vi "Rover_main.vi"() -> ()   [LabVIEW 2018]
uses:
  <vilib>/sound2/lvsound2.llb/Sound File Read Open.vi
  <vilib>/Instr/_visa.llb/VISA Configure Serial Port (Instr).vi
  <vilib>/Utility/file.llb/Write Delimited Spreadsheet (string).vi
  <vilib>/Utility/inputDevices.llb/keyboardAcquire.vi
  <vilib>/Utility/inputDevices.llb/closeKeyboard.vi
  <resource>/objmgr/imaqdx.rc
  <vilib>/vision/driver/NI_Vision_Acquisition_Software.lvlib
panel:
  out "DIS":dbl(knob) scale=0.0..500.0
  in  "Frames Per Second":u32=9
  out "Right view":bool
  out "Left view":bool
  out "Front view":bool
  in  "Camera port":refnum<k21>="cam5" caption="IMAQdx Session"
  in  "Video Modes":i32(listbox)
  out "Image":T1(plugin-control)
  out "AIR":dbl(knob) scale=500.0..1300.0
  out "Air Pressure Monitoring":string
  in  "path 3":path=path "C:/Users/向成/Desktop/ROVER PROJECT/LABVIEW codes/voice recognition/danger.wav" caption="路径"
  out "Voice recognition":bool
  in  "path":path=path "C:/Users/向成/Desktop/ROVER PROJECT/LABVIEW codes/voice recognition/activated.wav" caption="路径"
  in  "path 2":path=path "C:/Users/向成/Desktop/ROVER PROJECT/LABVIEW codes/voice recognition/failed.wav" caption="路径"
  out "Distance Monitoring":string
  in  "Sensors activation":bool
  out "TEM":dbl(slide) caption="量表" scale=0.0..50.0
  out "Temperature Monitoring":string
  out "gear":dbl(slide) scale=0.0..3.0
  out "LEFT":bool
  out "RIGHT":bool
  out "UP":bool
  out "DOWN":bool
  out "字符串监控":string
  in  "?":bool
  in  "Serial port":refnum<visa-resource-name>="COM4"
  # "Gear Stick Control"
  # "Motors Control"
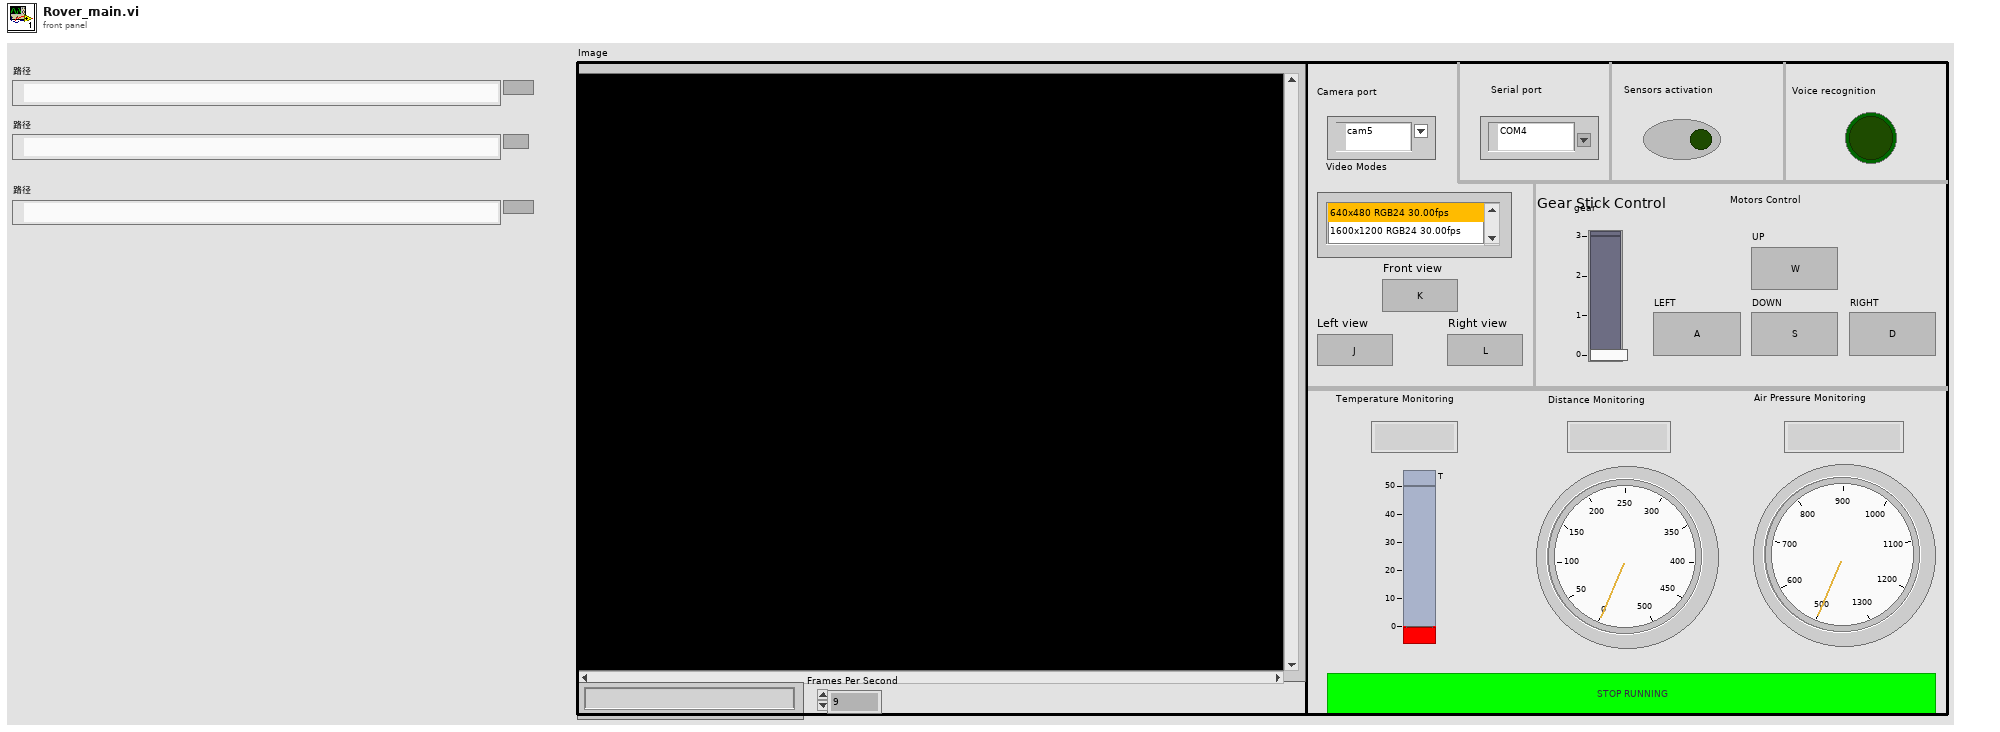
[diagram p1: front panel]
types:
  T1 = typedef "IMAQ Image.ctl" = refnum<image>
  T2 = enum16{"0", "1", "2", "3", "4", "5", "6", "7", "8", "9", "A", "B", "C", "D", "E", "F", "G", "H", "I", "J", "K", "L", "M", "N", "O", "P", "Q", "R", "S", "T", "U", "V", "W", "X", "Y", "Z", "F1", "F2", "F3", "F4", "F5", "F6", "F7", "F8", "F9", "F10", "F11", "F12", "F13", "F14", "F15", "ADD", "BACK", "BACKSLASH", "CAPITAL", "COMMA", "DECIMAL", "DELETE", "DIVIDE", "DOWN", "END", "EQUALS", "ESCAPE", "GRAVE (`)", "HOME", "INSERT", "LBRACKET", "LCONTROL", "LEFT", "L ALT", "LSHIFT", "LWIN", "MINUS", "MULTIPLY", "NEXT", "NUMLOCK", "NUMPAD_0", "NUMPAD_1", "NUMPAD_2", "NUMPAD_3", "NUMPAD_4", "NUMPAD_5", "NUMPAD_6", "NUMPAD_7", "NUMPAD_8", "NUMPAD_9", "PAUSE", "PERIOD", "PRIOR (PG UP)", "RBRACKET", "RCONTROL", "RETURN", "RIGHT", "R ALT", "RSHIFT", "RWIN", "SCROLL", "SEMICOLON", "SLASH", "SPACE", "SUBTRACT", "TAB", "UP", "ENTER (num pad)", "' (quote)"}
  T3 = typedef "Sound File Refnum.ctl" = refnum<file>
  T4 = enum32{"existing file", "new file", "new or existing file", "existing dir", "new dir", "new or existing dir", "existing file (use LLBs)", "new file (use LLBs)", "new or existing file (use LLBs)", "new or existing file or directory (use LLBs)"}
  T5 = typedef "IMAQdx.ctl" = refnum<k21>
  T6 = typedef "AviRefnum.ctl" = refnum<k1>
  T7 = enum16{"0", "1", "2", "3", "4", "5", "6", "7", "8", "9", "A", "B", "C", "D", "E", "F", "G", "H", "I", "J", "K", "L", "M", "N", "O", "P", "Q", "R", "S", "T", "U", "V", "W", "X", "Y", "Z", "F1", "F2", "F3", "F4", "F5", "F6", "F7", "F8", "F9", "F10", "F11", "F12", "F13", "F14", "F15", "ADD", "BACK", "BACKSLASH", "CAPITAL", "COMMA", "DECIMAL", "DELETE", "DIVIDE", "DOWN", "END", "EQUALS", "ESCAPE", "GRAVE (`)", "HOME", "INSERT", "LBRACKET", "LCONTROL", "LEFT", "L ALT", "LSHIFT", "LWIN", "MINUS", "MULTIPLY", "NEXT", "NUMLOCK", "NUMPAD_0", "NUMPAD_1", "NUMPAD_2", "NUMPAD_3", "NUMPAD_4", "NUMPAD_5", "NUMPAD_6", "NUMPAD_7", "NUMPAD_8", "NUMPAD_9", "PAUSE", "PERIOD", "PRIOR (PG UP)", "RBRACKET", "RCONTROL", "RETURN", "RIGHT", "R ALT", "RSHIFT", "RWIN", "SCROLL", "SEMICOLON", "SLASH", "SPACE", "SUBTRACT", "TAB", "UP", "ENTER (num pad)", "' (quote)"}[]
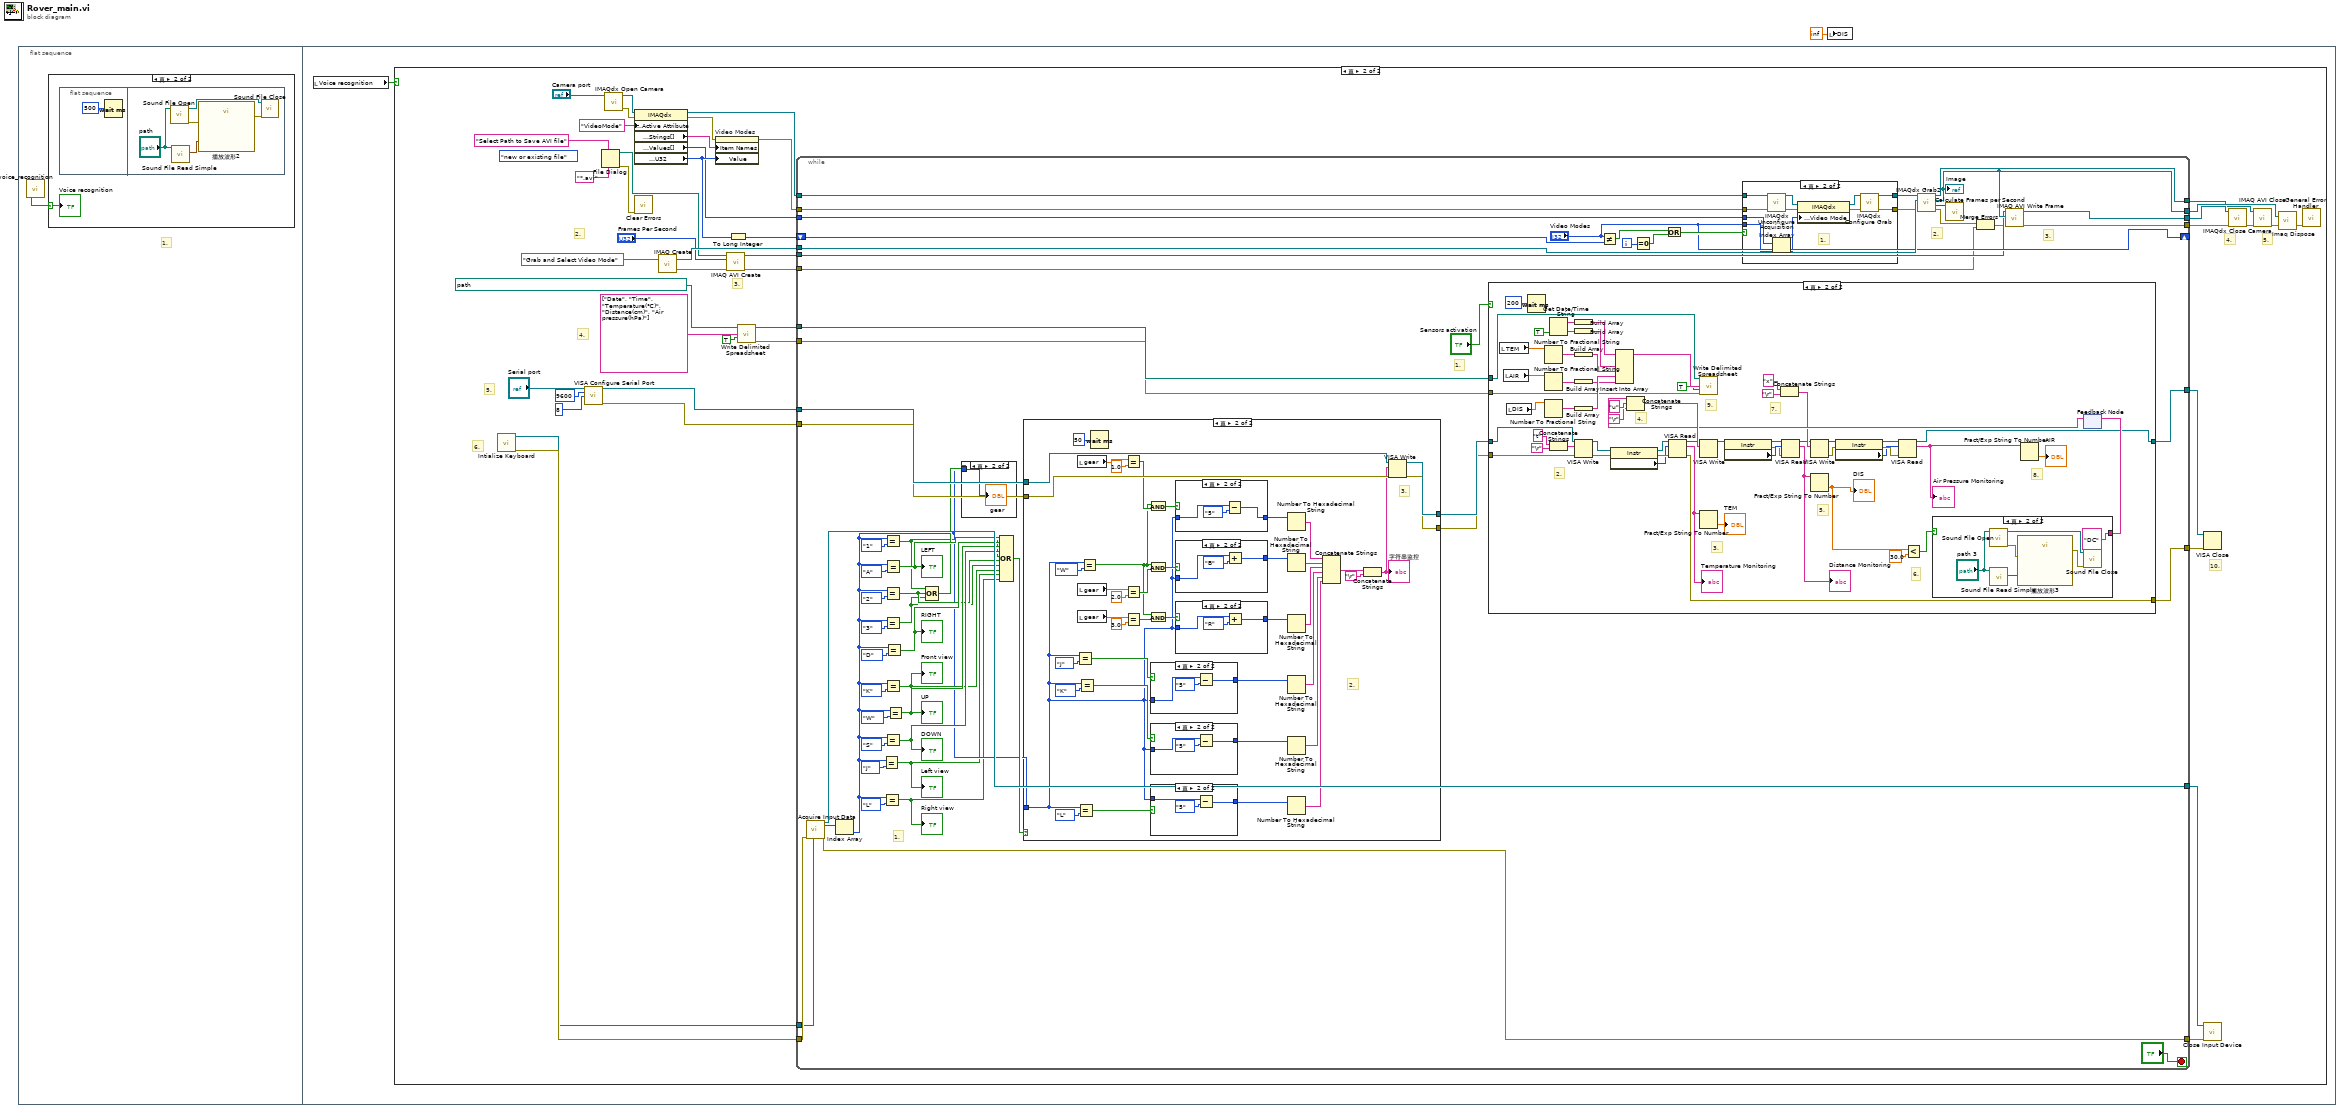
[diagram p0: block diagram]
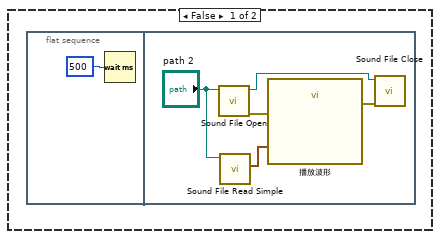
[diagram p2: hidden frame]
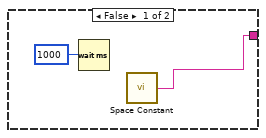
[diagram p6: hidden frame]
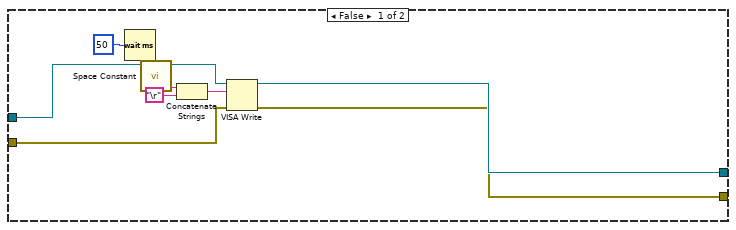
[diagram p8: hidden frame]
diagram:
  n1 = flat-sequence {
    frame #0 {
      # "1."
      n2 = call "voice_recognition.vi"() -> ("x < y?"=w2:bool)  [unwired: 5 in, 10 out]
      n3 = case shown="真" w2 {
        selector: w2 -> [_ w9]
        frame False {
          n4 = flat-sequence {
            frame #0 {
              n5 = Wait (ms)(milliseconds to wait=u32 500 ("等待时间（毫秒）")) -> ()  [unwired: 1 out]
            }
            frame #1 {
              n6 = call-poly <vilib>:"Sound File Open.vi"("path"="path 2") -> ("error out"=w5:errorcluster, "sound file refnum"=w7:T3)  [unwired: 9 in]
              n7 = call <vilib>:"Sound File Read Simple.vi"("path"="path 2") -> ("data"=w6:waveform(dbl)[])  [unwired: 7 in, 3 out]
              n8 = call "播放波形"("Data"=w6, "error in"=w5) -> ("error out"=w4:errorcluster)  [unwired: 17 in]
              n9 = call <vilib>:"Sound File Close.vi"("error in (no error)"=w4, "sound file refnum"=w7) -> ()  [unwired: 9 in, 1 out]
            }
          }
        }
        frame True {
          n10 = flat-sequence {
            frame #0 {
              n11 = Wait (ms)(milliseconds to wait=u32 500 ("等待时间（毫秒）")) -> ()  [unwired: 1 out]
            }
            frame #1 {
              n12 = call-poly <vilib>:"Sound File Open.vi"("path"="path") -> ("error out"=w13:errorcluster, "sound file refnum"=w11:T3)  [unwired: 9 in]
              n13 = call <vilib>:"Sound File Read Simple.vi"("path"="path") -> ("data"=w12:waveform(dbl)[])  [unwired: 7 in, 3 out]
              n14 = call "播放波形2"("Data"=w12, "error in"=w13) -> ("error out"=w14:errorcluster)  [unwired: 17 in]
              n15 = call <vilib>:"Sound File Close.vi"("error in (no error)"=w14, "sound file refnum"=w11) -> ()  [unwired: 9 in, 1 out]
            }
          }
          "Voice recognition" <- w9
        }
      }
    }
    frame #1 {
      n16 = local read "Voice recognition"() -> (w16:bool)
      n17 = case shown="真" w16 {
        frame False {
        }
        frame True {
          (unwired) T4."new or existing file" ("select mode (2)")
          # "10."
          # "5."
          # "4."
          # "6."
          # "3."
          # "5."
          # "4."
          # "2."
          n18 = call <vilib>:"Intialize Keyboard.vi"() -> ("error out"=w54:errorcluster, "device ID"=w53:refnum<k1>)  [unwired: 10 in]
          n19 = call-poly "VISA Configure Serial Port"("VISA resource name"="Serial port", "baud rate (9600)"=u32 9600, "data bits (8)"=u16 8) -> ("VISA resource name out"=w58:refnum<visa-resource-name>, "error out"=w59:errorcluster)  [unwired: 3 in, 8 out]
          n20 = File Dialog(6:"*.avi" ("pattern"), 7:"Select Path to Save AVI file" ("prompt")) -> (0:w18:errorcluster, 3:w19:path)  [unwired: 1 in, 6 out]
          n21 = call <vilib>:"IMAQdx Open Camera.vi"("Session In"="Camera port") -> ("error out"=w47:errorcluster, "Session Out"=w46:T5)  [unwired: 2 in, 7 out]
          n22 = property class="IMAQdx"(reference=w46, error in=w47, "Camera Attributes:Active Attribute"="VideoMode" ("ActiveAttribute")) -> (reference out=w40:T5, error out=w48:errorcluster, "Camera Attributes:Enum:Strings[]"=w49:string[], "Camera Attributes:Enum:Values[]"=w42:u32[], "Camera Attributes:Value:U32"=w50:u32)
          n23 = call <vilib>:"Clear Errors.vi"("error in (no error)"=w18) -> ()  [unwired: 5 in, 2 out]
          n24 = call "IMAQ Create"("Image Name"="Grab and Select Video Mode") -> ("New Image"=w41:T1, "error out"=w24:errorcluster)  [unwired: 3 in, 1 out]
          n25 = property on="Video Modes" class="LstBox (严格)"(error in=w48, "Item Names"=w49, "Value"=w50) -> (error out=w25:errorcluster)  [unwired: 1 in, 1 out]
          n26 = call "IMAQ AVI Create"("error in (no error)"=w24, "Frames Per Second"="Frames Per Second", "AVI Path"=w19) -> ("error out"=w17:errorcluster, "Avi Refnum"=w23:T6)  [unwired: 4 in, 3 out]
          n27 = To Long Integer(number=w50) -> (32bit integer=w39:i32)
          n28 = call-poly <vilib>:"Write Delimited Spreadsheet.vi"("file path (dialog if empty)"=path "C:/Users/向成/Desktop/rover_project/Data_Storage/data_acquired", "1D data"=string[] ["Date", "Time", "Temperature(℃)", "Distance(cm)", "Air pressure(hPa)"], "append to file? (new file:F)"=TRUE) -> ("new file path (Not A Path if cancelled)"=w31:path, "error out"=w30:errorcluster)  [unwired: 11 in]
          n29 = while {
            tunnel: w53 -> [w118]
            tunnel: w54 -> [w119]
            tunnel: w58 -> [w116]
            tunnel: w59 -> [w115]
            tunnel: [w117] -> w56
            tunnel: [w114] -> w57
            tunnel: [w96] -> w60
            tunnel: w42 -> [w93]
            tunnel: w41 -> [w92]
            tunnel: w40 -> [w91]
            shift-right: ["Video Modes"] -> _
            shift-left: w39 -> [w83]
            tunnel: [w67] -> w37
            tunnel: [w64] -> w36
            tunnel: [w82] -> w35
            tunnel: w31 -> [w71]
            tunnel: w30 -> [w70]
            tunnel: [w69] -> w29
            tunnel: w25 -> [w68]
            tunnel: [w66] -> w28
            tunnel: w23 -> [w65]
            tunnel: w17 -> [w62]
            i -> [w81]
            stop <- "?" stop-if-true
            # "1."
            # "3."
            # "2."
            # "1."
            n30 = call-poly <vilib>:"Acquire Input Data.vi"("device ID"=w118, "error in (no error)"=w119) -> ("device ID"=w117:refnum<k1>, "keys pressed"=w111:T7, "error out"=w114:errorcluster)  [unwired: 15 in]
            n31 = Index Array(array=w111) -> (element=w75:T2)  [unwired: 1 in]
            n32 = Equal?(x=w75, y=T2."J") -> (x = y?=w74:bool)
            "Left view" <- w74
            n33 = Equal?(x=w75, y=T2."L") -> (x = y?=w73:bool)
            "Right view" <- w73
            n34 = Equal?(x=w75, y=T2."1") -> (x = y?=w99:bool)
            n35 = Equal?(x=w75, y=T2."2") -> (x = y?=w98:bool)
            n36 = Equal?(x=w75, y=T2."3") -> (x = y?=w97:bool)
            n37 = Equal?(x=w75, y=T2."S") -> (x = y?=w101:bool)
            "DOWN" <- w101
            n38 = Equal?(x=w75, y=T2."A") -> (x = y?=w104:bool)
            "LEFT" <- w104
            n39 = Equal?(x=w75, y=T2."K") -> (x = y?=w78:bool)
            "Front view" <- w78
            n40 = Equal?(x=w75, y=T2."D") -> (x = y?=w103:bool)
            "RIGHT" <- w103
            n41 = Equal?(x=w75, y=T2."W") -> (x = y?=w102:bool)
            "UP" <- w102
            n42 = Compound Arithmetic op=OR ("复合运算")(w99, w98, w97) -> (w100:bool)
            n43 = case shown="真" w100 {
              tunnel: w75 -> [_ w201]
              frame False {
              }
              frame True {
                "gear" <- w201
              }
            }
            n44 = Compound Arithmetic op=OR ("复合运算")(w104, w103, w102, w101, w99, w98, w97, w78, w74, w73) -> (w110:bool)
            n45 = case shown="真" w110 {
              tunnel: [w204 w249] -> w95
              tunnel: [w203 w248] -> w94
              tunnel: w75 -> [_ w213]
              tunnel: w116 -> [w205 w247]
              tunnel: w115 -> [w206 w246]
              frame False {
                n46 = Wait (ms)(milliseconds to wait=u32 50 ("等待时间（毫秒）")) -> ()  [unwired: 1 out]
                n47 = call <vilib>:"Space Constant.vi"() -> ("String"=w207:string)
                n48 = Concatenate Strings(w207, "\r") -> (w209:string)
                n49 = VISA Write(VISA resource name=w205, write buffer=w209, error in (no error)=w206) -> (VISA resource name out=w204:refnum<visa-resource-name>, error out=w203:errorcluster)  [unwired: 1 out]
              }
              frame True {
                # "3."
                # "2."
                n50 = Equal?(x=w213, y=T2."J") -> (x = y?=w219:bool)
                n51 = Equal?(x=w213, y=T2."L") -> (x = y?=w217:bool)
                n52 = local read "gear"() -> (w244:dbl)
                n53 = local read "gear"() -> (w238:dbl)
                n54 = local read "gear"() -> (w233:dbl)
                n55 = Equal?(x=w213, y=T2."K") -> (x = y?=w218:bool)
                n56 = Equal?(x=w213, y=T2."W") -> (x = y?=w225:bool)
                n57 = Wait (ms)(milliseconds to wait=u32 50 ("等待时间（毫秒）")) -> ()  [unwired: 1 out]
                n58 = Equal?(x=w244, y=1.0) -> (x = y?=w242:bool)
                n59 = Equal?(x=w238, y=2.0) -> (x = y?=w236:bool)
                n60 = Equal?(x=w233, y=3.0) -> (x = y?=w234:bool)
                n61 = And(x=w225, y=w242) -> (x .and. y?=w241:bool)
                n62 = And(x=w225, y=w236) -> (x .and. y?=w240:bool)
                n63 = And(x=w225, y=w234) -> (x .and. y?=w226:bool)
                n64 = case shown="真" w219 {
                  tunnel: [_ w258] -> w216
                  tunnel: w213 -> [_ w257]
                  frame False {
                  }
                  frame True {
                    n65 = Subtract(x=w257, y=T2."5") -> (x-y=w258:u16)
                  }
                }
                n66 = case shown="真" w218 {
                  tunnel: [_ w255] -> w215
                  tunnel: w213 -> [_ w254]
                  frame False {
                  }
                  frame True {
                    n67 = Subtract(x=w254, y=T2."5") -> (x-y=w255:u16)
                  }
                }
                n68 = case shown="真" w217 {
                  tunnel: [_ w252] -> w214
                  tunnel: w213 -> [_ w251]
                  frame False {
                  }
                  frame True {
                    n69 = Subtract(x=w251, y=T2."5") -> (x-y=w252:u16)
                  }
                }
                n70 = case shown="真" w241 {
                  tunnel: w213 -> [w266 w269]
                  tunnel: [w266 w267] -> w239
                  frame False {
                  }
                  frame True {
                    n71 = Subtract(x=w269, y=T2."5") -> (x-y=w267:u16)
                  }
                }
                n72 = case shown="真" w240 {
                  tunnel: [_ w264] -> w232
                  tunnel: w213 -> [_ w263]
                  frame False {
                  }
                  frame True {
                    n73 = Add(x=w263, y=T2."B") -> (x+y=w264:u16)
                  }
                }
                n74 = case shown="真" w226 {
                  tunnel: [_ w261] -> w229
                  tunnel: w213 -> [_ w260]
                  frame False {
                  }
                  frame True {
                    n75 = Add(x=w260, y=T2."R") -> (x+y=w261:u16)
                  }
                }
                n76 = Number To Hexadecimal String(2:w239) -> (0:w230:string)  [unwired: 1 in]
                n77 = Number To Hexadecimal String(2:w232) -> (0:w231:string)  [unwired: 1 in]
                n78 = Number To Hexadecimal String(2:w229) -> (0:w228:string)  [unwired: 1 in]
                n79 = Number To Hexadecimal String(2:w216) -> (0:w212:string)  [unwired: 1 in]
                n80 = Number To Hexadecimal String(2:w215) -> (0:w210:string)  [unwired: 1 in]
                n81 = Number To Hexadecimal String(2:w214) -> (0:w211:string)  [unwired: 1 in]
                n82 = Concatenate Strings(w230, w231, w228, w212, w210, w211) -> (w227:string)
                n83 = Concatenate Strings(w227, "\r") -> (w224:string)
                "字符串监控" <- w224
                n84 = VISA Write(VISA resource name=w247, write buffer=w224, error in (no error)=w246) -> (VISA resource name out=w249:refnum<visa-resource-name>, error out=w248:errorcluster)  [unwired: 1 out]
              }
            }
            n85 = case shown="真" "Sensors activation" {
              tunnel: [w134 w192] -> w96
              tunnel: w95 -> [w133 w191]
              tunnel: w94 -> [w134 w190]
              tunnel: w71 -> [_ w175]
              tunnel: w70 -> [_ w173]
              tunnel: [w133 w137] -> w69
              frame False {
              }
              frame True {
                # "8."
                # "7."
                # "4."
                # "6."
                # "5."
                # "3."
                # "2."
                # "9."
                n86 = local read "TEM"() -> (w189:dbl)
                n87 = local read "AIR"() -> (w187:dbl)
                n88 = local read "DIS"() -> (w135:dbl)
                n89 = Wait (ms)(milliseconds to wait=u32 200 ("等待时间（毫秒）")) -> ()  [unwired: 1 out]
                n90 = Number To Fractional String(number=w189) -> (F-format string=w188:string)  [unwired: 3 in]
                n91 = Number To Fractional String(number=w187) -> (F-format string=w186:string)  [unwired: 3 in]
                n92 = Number To Fractional String(number=w135) -> (F-format string=w185:string)  [unwired: 3 in]
                n93 = Get Date/Time String(want seconds? (F)=TRUE ("需要秒？(F)")) -> (date string=w179:string, time string=w180:string)  [unwired: 2 in]
                n94 = Concatenate Strings("t" ("字符串"), "\r") -> (w167:string)
                n95 = Build Array(w179) -> (w181:string[])
                n96 = Build Array(w180) -> (w182:string[])
                n97 = Build Array(w188) -> (w184:string[])
                n98 = Build Array(w186) -> (w177:string[])
                n99 = Build Array(w185) -> (w178:string[])
                n100 = VISA Write(VISA resource name=w191, write buffer=w167, error in (no error)=w190) -> (VISA resource name out=w169:refnum<visa-resource-name>, error out=w168:errorcluster)  [unwired: 1 out]
                n101 = property class="Instr"(reference=w169, error in=w168) -> (reference out=w172:refnum<visa-resource-name>, error out=w171:errorcluster, "Serial Settings:Number of Bytes at Serial Port"=w170:u32)
                n102 = Insert Into Array(array=w181, new element #1=w182, new element #2=w184, new element #3=w178, new element #4=w177) -> (w183:string[])  [unwired: 1 in]
                n103 = VISA Read(VISA resource name=w172, byte count=w170, error in (no error)=w171) -> (VISA resource name out=w154:refnum<visa-resource-name>, read buffer=w162:string, error out=w192:errorcluster)  [unwired: 1 out]
                "Temperature Monitoring" <- w162
                n104 = call-poly <vilib>:"Write Delimited Spreadsheet.vi"("file path (dialog if empty)"=w175, "1D data"=w183, "append to file? (new file:F)"=TRUE, "error in (no error)"=w173) -> ()  [unwired: 10 in, 2 out]
                n105 = Fract/Exp String To Number(string=w162) -> (number=→"TEM":dbl)  [unwired: 3 in, 1 out]
                n106 = Concatenate Strings("x" ("字符串"), "\r") -> (w143:string)
                n107 = feedback #1() -> (w149:string)  [unwired: 1 in]
                n108 = Concatenate Strings(w149, "u" ("字符串"), "\r") -> (w159:string)
                n109 = VISA Write(VISA resource name=w154, write buffer=w159) -> (VISA resource name out=w155:refnum<visa-resource-name>)  [unwired: 1 in, 2 out]
                n110 = property class="Instr"(reference=w155) -> (reference out=w156:refnum<visa-resource-name>, error out=w157:errorcluster, "Serial Settings:Number of Bytes at Serial Port"=w158:u32)  [unwired: 1 in]
                n111 = VISA Read(VISA resource name=w156, byte count=w158, error in (no error)=w157) -> (VISA resource name out=w139:refnum<visa-resource-name>, read buffer=w150:string)  [unwired: 2 out]
                "Distance Monitoring" <- w150
                n112 = VISA Write(VISA resource name=w139, write buffer=w143) -> (VISA resource name out=w145:refnum<visa-resource-name>, error out=w144:errorcluster)  [unwired: 1 in, 1 out]
                n113 = Fract/Exp String To Number(string=w150) -> (number=w136:dbl)  [unwired: 3 in, 1 out]
                "DIS" <- w136
                n114 = property class="Instr"(reference=w145, error in=w144) -> (reference out=w148:refnum<visa-resource-name>, error out=w147:errorcluster, "Serial Settings:Number of Bytes at Serial Port"=w146:u32)
                n115 = VISA Read(VISA resource name=w148, byte count=w146, error in (no error)=w147) -> (VISA resource name out=w137:refnum<visa-resource-name>, read buffer=w138:string)  [unwired: 2 out]
                "Air Pressure Monitoring" <- w138
                n116 = Less?(x=w136, y=30.0) -> (x < y?=w153:bool)
                n117 = case shown="真" w153 {
                  tunnel: [w193 "DC" ("字符串")] -> w151
                  frame False {
                    n118 = Wait (ms)(milliseconds to wait=u32 1000 ("等待时间（毫秒）")) -> ()  [unwired: 1 out]
                    n119 = call <vilib>:"Space Constant.vi"() -> ("String"=w193:string)
                  }
                  frame True {
                    n120 = call-poly <vilib>:"Sound File Open.vi"("path"="path 3") -> ("error out"=w197:errorcluster, "sound file refnum"=w195:T3)  [unwired: 9 in]
                    n121 = call <vilib>:"Sound File Read Simple.vi"("path"="path 3") -> ("data"=w196:waveform(dbl)[])  [unwired: 7 in, 3 out]
                    n122 = call "播放波形3"("Data"=w196, "error in"=w197) -> ("error out"=w198:errorcluster)  [unwired: 17 in]
                    n123 = call <vilib>:"Sound File Close.vi"("error in (no error)"=w198, "sound file refnum"=w195) -> ()  [unwired: 9 in, 1 out]
                  }
                }
                n124 = Fract/Exp String To Number(string=w138) -> (number=→"AIR":dbl)  [unwired: 3 in, 1 out]
                n125 = feedback-in #1(w151) -> ()
              }
            }
            n126 = Not Equal?(x="Video Modes", y=w83) -> (x != y?=w89:bool)
            n127 = Equal To 0?(x=w81) -> (x = 0?=w88:bool)
            n128 = Or(x=w89, y=w88) -> (x .or. y?=w90:bool)
            n129 = case shown="真" w90 {
              tunnel: w91 -> [w121 w130]
              tunnel: w68 -> [w120 w129]
              tunnel: [w121 w126] -> w86
              tunnel: [w120 w127] -> w87
              tunnel: w93 -> [_ w132]
              tunnel: "Video Modes" -> [_ w131]
              frame False {
              }
              frame True {
                # "1."
                n130 = call <vilib>:"IMAQdx Unconfigure Acquisition.vi"("error in"=w129, "Session In"=w130) -> ("error out"=w123:errorcluster, "Session Out"=w128:T5)  [unwired: 8 out]
                n131 = Index Array(array=w132, index=w131) -> (element=w122:u32)
                n132 = property class="IMAQdx"(reference=w128, error in=w123, "Acquisition Attributes:Video Mode"=w122) -> (reference out=w125:T5, error out=w124:errorcluster)
                n133 = call <vilib>:"IMAQdx Configure Grab.vi"("error in"=w124, "Session In"=w125) -> ("error out"=w127:errorcluster, "Session Out"=w126:T5)  [unwired: 1 in, 7 out]
              }
            }
            n134 = call <vilib>:"IMAQdx Grab2.vi"("error in"=w87, "Image In"=w92, "Session In"=w86) -> ("error out"=w63:errorcluster, "Buffer Number Out"=w85:u32, "Image Out"=w67:T1, "Session Out"=w82:T5)  [unwired: 5 in]
            "Image" <- w67
            n135 = call <vilib>:"Calculate Frames per Second.vi"("Buffer Number"=w85) -> ()  [unwired: 8 in, 3 out]
            n136 = Merge Errors(w63, w62) -> (w61:errorcluster)
            n137 = call "IMAQ AVI Write Frame"("error in (no error)"=w61, "Image"=w67, "Avi Refnum"=w65) -> ("error out"=w64:errorcluster, "Avi Refnum (duplicate)"=w66:T6)  [unwired: 1 in, 6 out]
          }
          n138 = VISA Close(VISA resource name=w29, error in (no error)=w60) -> ()  [unwired: 1 out]
          n139 = call-poly <vilib>:"Close Input Device.vi"("error in (no error)"=w57, "device ID"=w56) -> ()  [unwired: 8 in, 1 out]
          n140 = call <vilib>:"IMAQdx Close Camera.vi"("error in"=w36, "Session In"=w35) -> ("error out"=w27:errorcluster)  [unwired: 9 out]
          n141 = call "IMAQ AVI Close"("error in (no error)"=w27, "Avi Refnum"=w28) -> ("error out"=w26:errorcluster)  [unwired: 9 out]
          n142 = call "Imaq Dispose"("Image"=w37, "error in (no error)"=w26) -> ("error out"=w38:errorcluster)  [unwired: 4 in]
          n143 = call <vilib>:"General Error Handler.vi"("error in (no error)"=w38) -> ()  [unwired: 2 in, 13 out]
        }
      }
    }
  }
  n144 = local write "DIS"(inf ("DIS")) -> ()
